vi "DFD FXP Simulation.vi"   [LabVIEW 2017, in "NI_DigFilterLicensed.lvlib"]
doc: "Simulates the filtering process continuously and generates a filtering statistics report for a fixed-point filter. The data type you wire to the <B>signal in</B> input determines the polymorphic instance to use."
uses:
  <vilib>/addons/Digital Filter Design/NI_DigFilterLicensed.lvlib
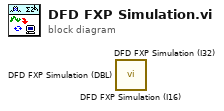
[diagram p0: block diagram]
diagram:
  n1 = call <vilib>:"DFD FXP Simulation (I16).vi"() -> ()  [unwired: 8 in, 4 out]
  n2 = call <vilib>:"DFD FXP Simulation (I32).vi"() -> ()  [unwired: 8 in, 4 out]
  n3 = call <vilib>:"DFD FXP Simulation (DBL).vi"() -> ()  [unwired: 8 in, 4 out]
